vi "Build Tx Generic Engine Configuration.vi"(8 "error in":errorcluster, 9 "port properties":T1, 10 "board properties":T2 {"portConfig" items=["FDX_SINGLE", "FDX_REDUNDANT"]; "portSpeed" items=["FDX_100MBIT", "FDX_10MBIT", "FDX_AUTO_100MBIT", "FDX_AUTO_10MBIT", "FDX_AUTO_ERROR", "FDX_1000MBIT"]}, 11 "section ref in":T9=18446744073709551615 format="%.0x") -> (0 "error out":errorcluster, 2 "Tx cluster out":T3 {"channel settings"."Payload Parameter Array"."Parameters"."encoding" items=["BNR", "BCD", "Discrete"]}, 3 "section ref out":T9 format="%.0x")   [LabVIEW 2020, in "AIM ARINC 664 Scripting.lvlib"]
uses:
  AIM ARINC 664 Scripting.lvlib
  <vilib>/NI VeriStand/Custom Device API/Custom Device Item Ref.ctl
  Shared/hardware_channels_tx.ctl
  Shared/channel_settings_tx.ctl
  Shared/Frame Payload Parameters.ctl
  Shared/Encoding (Arinc664).ctl
  Shared/RawFrame_entry.ctl
  <instrlib>/AIM GmbH/_AIM 664/_controls/queue_header_generic.ctl
  Import/_typedefs/board_setup.ctl
  Import/_typedefs/port_setup.ctl
  Import/_typedefs/tx_generic_setup.ctl
  Import/AIM ARINC 664 Import.lvlib
  <instrlib>/AIM GmbH/_AIM 664/AIM664LV.lvlib
  <vilib>/NI VeriStand/Custom Device API/Custom Device API.lvlib
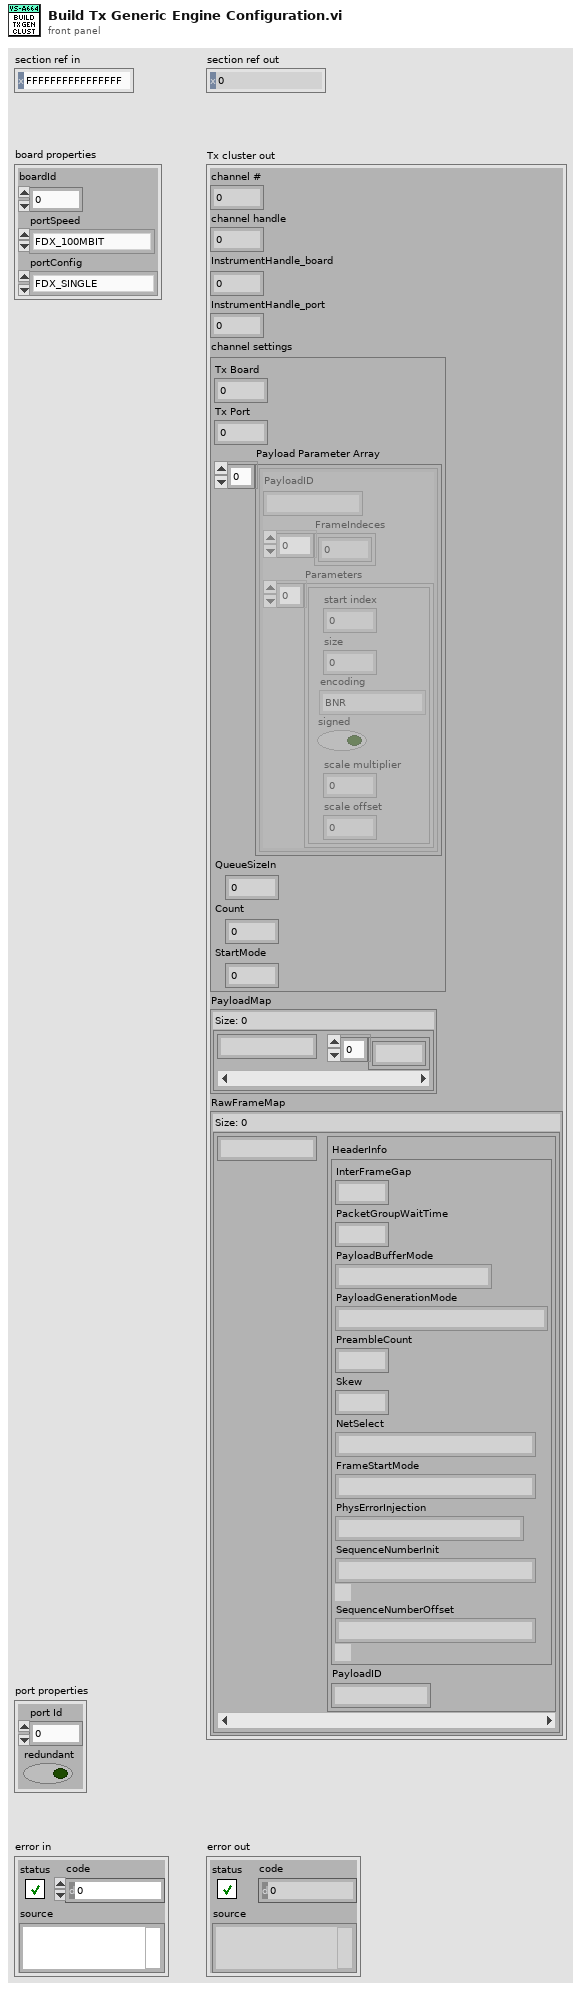
[diagram p1: front panel]
types:
  T1 = typedef "AIM ARINC 664 Import.lvlib/port_setup.ctl" = cluster{"port Id":u32, "redundant":bool}
  T2 = typedef "AIM ARINC 664 Import.lvlib/board_setup.ctl" = cluster{"boardId":u32, "portSpeed":u32, "portConfig":u32}
  T3 = typedef "hardware_channels_tx.ctl" = cluster{"channel #":u16, "channel handle":u64, "InstrumentHandle_board":u32, "InstrumentHandle_port":u32, "channel settings":T4, "PayloadMap":map{string, u8[]}, "RawFrameMap":map{string, T7}}
  T4 = typedef "channel_settings_tx.ctl" = cluster{"Tx Board":u32, "Tx Port":u32, "Payload Parameter Array":T5[], "QueueSizeIn":u32, "Count":u32, "StartMode":u32}
  T5 = typedef "Frame Payload Parameters.ctl" = cluster{"PayloadID":string, "FrameIndeces":u32[], "Parameters":cluster{"start index":i32, "size":i32, "encoding":T6, "signed":bool, "scale multiplier":dbl, "scale offset":dbl}[]}
  T6 = typedef "Encoding (Arinc664).ctl" = u16
  T7 = typedef "RawFrame_entry.ctl" = cluster{"HeaderInfo":T8, "PayloadID":string}
  T8 = typedef "AIM664LV.lvlib/queue_header_generic.ctl" = cluster{"InterFrameGap":u32, "PacketGroupWaitTime":u32, "PayloadBufferMode":u8, "PayloadGenerationMode":u8, "PreambleCount":u8, "Skew":u32, "NetSelect":u8, "FrameStartMode":u8, "PhysErrorInjection":u32, "SequenceNumberInit":u16, "SequenceNumberOffset":u16}
  T9 = typedef "Custom Device API.lvlib/Custom Device Item Ref.ctl" = u64
  T10 = typedef "AIM ARINC 664 Import.lvlib/tx_generic_setup.ctl" = cluster{"QueueSizeIn":u32, "Count":i32, "StartMode":i32}
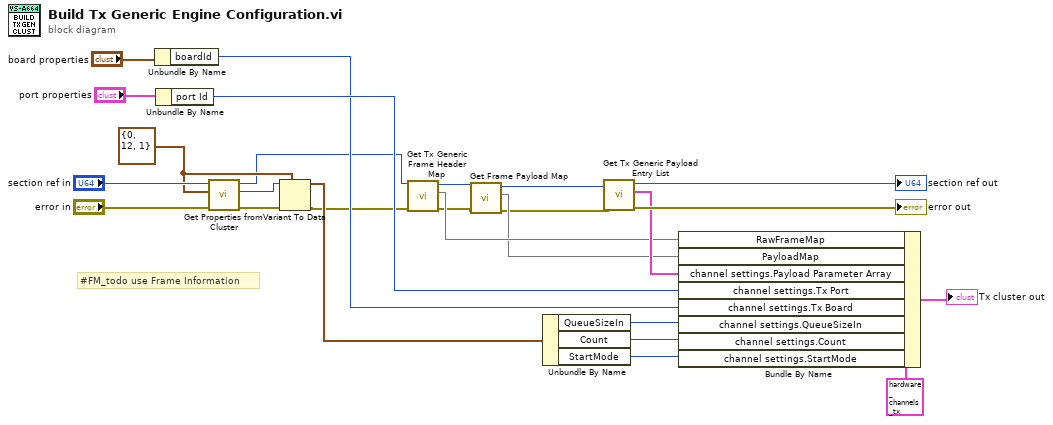
[diagram p0: block diagram]
diagram:
  w9 = T10 {"QueueSizeIn"=0, "Count"=12, "StartMode"=1} ("tx_generic_setup")
  # "#FM_todo use Frame Information"
  n1 = Unbundle By Name("board properties") -> ("boardId"=w12:u32)
  n2 = Unbundle By Name("port properties") -> ("port Id"=w14:u32)
  n3 = call "Get Properties from Cluster.vi"("error in"="error in", "Variant Cluster"=w9, "custom device ref in"="section ref in") -> ("error out"=w19:errorcluster, "data"=w20:variant, "custom device ref out"=w8:T9)  [unwired: 5 in, 1 out]
  n4 = Variant To Data(error in=w19, type=w9, Variant=w20) -> (data=w10:T10, error out=w7:errorcluster)
  n5 = call "Get Tx Generic Frame Header Map.vi"("error in"=w7, "custom device ref in"=w8) -> ("error out"=w2:errorcluster, "Raw Frame Header Map"=w6:map{string, T7}, "custom device ref out"=w5:T9)  [unwired: 7 in]
  n6 = call "Get Frame Payload Map.vi"("error in"=w2, "custom device ref in"=w5) -> ("error out"=w1:errorcluster, "Payload Map"=w3:map{string, u8[]}, "custom device ref out"=w4:T9)  [unwired: 7 in]
  n7 = Unbundle By Name(w10) -> ("QueueSizeIn"=w16:u32, "Count"=w17:i32, "StartMode"=w18:i32)
  n8 = call "Get Tx Generic Payload Entry List.vi"("error in"=w1, "custom device ref in"=w4) -> ("error out"=→"error out":errorcluster, "Payload Entry List"=w21:T5[], "custom device ref out"=→"section ref out":T9)  [unwired: 6 in, 1 out]
  n9 = Bundle By Name(cluster=T3 {"channel #"=0, "channel handle"=0, "InstrumentHandle_board"=0, "InstrumentHandle_port"=0, "channel settings"={"Tx Board"=0, "Tx Port"=0, "Payload Parameter Array"=[{"PayloadID"="", "FrameIndeces"=[], "Parameters"=[]}, {"PayloadID"="", "FrameIndeces"=[], "Parameters"=[]}], "QueueSizeIn"=0, "Count"=0, "StartMode"=0}, "PayloadMap"={}, "RawFrameMap"={}} ("TX Parameters"), "RawFrameMap"=w6, "PayloadMap"=w3, "channel settings.Payload Parameter Array"=w21, "channel settings.Tx Port"=w14, "channel settings.Tx Board"=w12, "channel settings.QueueSizeIn"=w16, "channel settings.Count"=w17, "channel settings.StartMode"=w18) -> (→"Tx cluster out":T3)
